vi "Read DBL Configuration.vi"(8 "error in (no error)":errorcluster, 9 "Default If Not Found":dbl=nan, 10 "Name":string, 11 "database-configuration in":refnum<class "configuration-database.lvclass">) -> (0 "error out":errorcluster, 1 "Not Found?":bool, 2 "Value":dbl, 3 "database-configuration out":refnum<class "configuration-database.lvclass">)   [LabVIEW 2020, in "configuration-database.lvlib" / "configuration-database.lvclass"]
uses:
  configuration-database.lvclass
  configuration-database.lvclass/configuration-database.ctl
  25c4a073-bb0f-4582-bca8-bdab031859cb.vi
  25c4a073-bb0f-4582-bca8-bdab031859cb.vi/5136a74e-d4d9-4a1b-b735-d1b214723075.vi
  <vilib>/Utility/error.llb/Error Cluster From Error Code.vi
  IConfigDBQueries/IConfigurationDatabaseQueries.lvclass
  externals/database-interface/IDatabase/IDatabase/IDatabase.lvclass
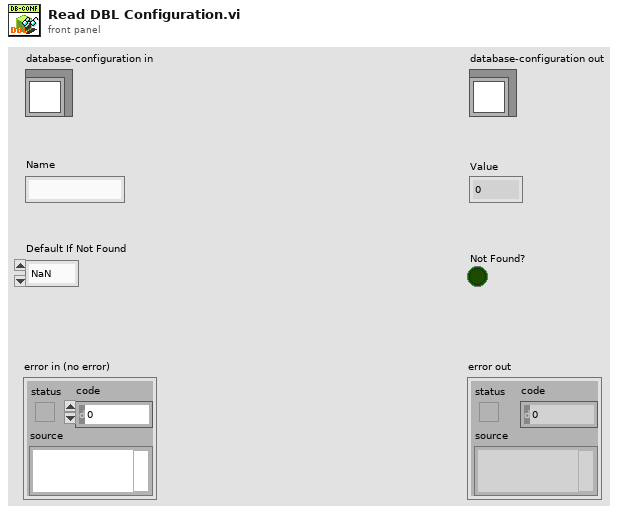
[diagram p1: front panel]
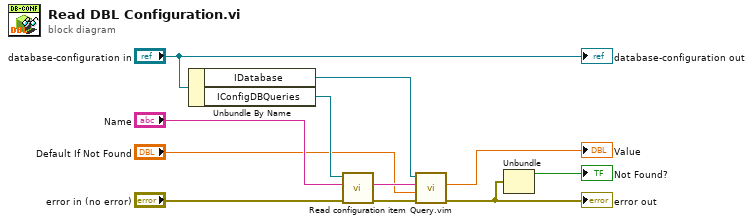
[diagram p0: block diagram]
diagram:
  n1 = Unbundle By Name("database-configuration in") -> ("IDatabase"=w7:refnum<class "IDatabase.lvclass">, "IConfigDBQueries"=w10:refnum<class "IConfigurationDatabaseQueries.lvclass">)
  n2 = call-dynamic "Read configuration item.vi"("error in (no error)"="error in (no error)", "configuration item"="Name", "IConfigDBQueries in"=w10) -> ("error out"=w6:errorcluster, "result"=w5:string)  [unwired: 7 in]
  n3 = call "Query.vim"("error in (no error)"=w6, "Type and Default"="Default If Not Found", "Query string"=w5, "IDatabase in"=w7) -> ("error out"=w2:errorcluster, "Result"=→"Value":dbl)  [unwired: 5 in, 1 out]
  "error out" <- w2
  n4 = Unbundle(w2) -> ("status"=→"Not Found?":bool)  [unwired: 2 out]
  "database-configuration out" <- "database-configuration in"
